vi "Default PWM Channels.vi"(1 "Channels":T3={"# Input Channels"=0, "# Output Channels"=0, "Channel Type"=enum."Digital", "Units"=""}) -> (0 "PWM":T1 {"PWM Channels"."PWM frequency" items=["1 Hz", "50 Hz", "250 Hz", "500 Hz", "1 kHz", "5 kHz", "10 kHz", "20 kHz"]})   [LabVIEW 2020, in "Modules.lvlib" / "SD Module.lvclass"]
uses:
  SD Module.lvclass
  RSI Module/Channels.ctl
  RSI Module/Channel Type.ctl
  Type Defs/PWM.ctl
  Type Defs/PWM Channel.ctl
  RSI Module/RSI Module.lvclass
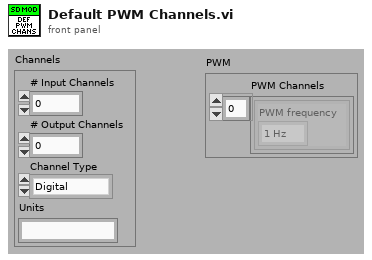
[diagram p1: front panel]
types:
  T1 = typedef "Modules.lvlib/SD Module.lvclass/PWM.ctl" = cluster{"PWM Channels":T2[]}
  T2 = typedef "Modules.lvlib/SD Module.lvclass/PWM Channel.ctl" = cluster{"PWM frequency":u32}
  T3 = typedef "Modules.lvlib/RSI Module.lvclass/Channels.ctl" = cluster{"# Input Channels":i32, "# Output Channels":i32, "Channel Type":T4, "Units":string}
  T4 = typedef "Modules.lvlib/RSI Module.lvclass/Channel Type.ctl" = enum16{"Analog", "Digital"}
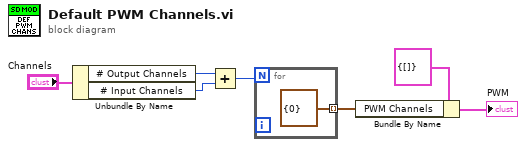
[diagram p0: block diagram]
diagram:
  n1 = Unbundle By Name("Channels") -> ("# Output Channels"=w1:i32, "# Input Channels"=w2:i32)
  n2 = Add(x=w1, y=w2) -> (x+y=w3:i32)
  n3 = for {
    N: w3 -> [_]
    tunnel: [T2 {"PWM frequency"=0} ("PWM Channel")] -> w7 mode=indexing
  }
  n4 = Bundle By Name(cluster=T1 {"PWM Channels"=[]} ("PWM"), "PWM Channels"=w7) -> (→"PWM":T1)
